vi "SetStringValue.vi"(8 "error in (no error)":errorcluster caption="错误输入（无错误）", 9 "strValue":string, 10 "strKey":string, 11 "handle":u64) -> (0 "error out":errorcluster caption="错误输出", 1 "strValue":string, 2 "function return":i32, 3 "handle out":u64)   [LabVIEW 2015, in "MvCameraControl.lvlib"]
doc: "MV_LV_API int __stdcall GetStringValue( void* handle, const char* strKey, MVCC_STRINGVALUE *pStringValue);"
uses:
  MvCameraControl.lvlib
  MvCameraControl.dll
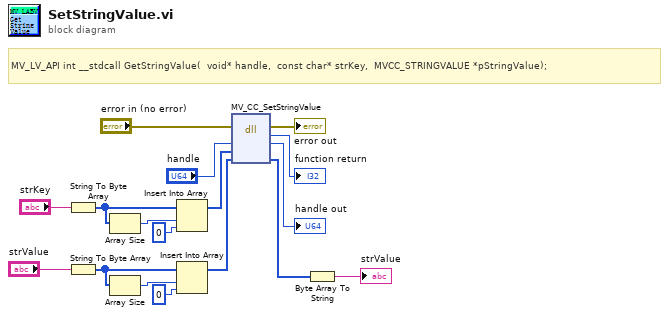
[diagram p0: block diagram]
diagram:
  # "MV_LV_API int __stdcall GetStringValue(  void* handle,  const char* strKey,  MVCC_STRINGVALUE *pStringValue);"
  n1 = String To Byte Array(string="strKey") -> (unsigned byte array=w13:u8[])
  n2 = String To Byte Array(string="strValue") -> (unsigned byte array=w8:u8[])
  n3 = Array Size(array=w13) -> (size(s)=w12:i32)
  n4 = Array Size(array=w8) -> (size(s)=w7:i32)
  n5 = Insert Into Array(array=w13, index=w12, new element=u8 0 ("新元素/子数组")) -> (w9:u8[])
  n6 = Insert Into Array(array=w8, index=w7, new element=u8 0 ("新元素/子数组")) -> (w4:u8[])
  n7 = dll-call lib="MvCameraControl.dll" fn="MV_CC_SetStringValue"(error in="error in (no error)", "handle"="handle", "strKey"=w9, "pStringValue"=w4) -> (error out=→"error out":errorcluster, "返回类型"=→"function return":i32, "handle"=→"handle out":u64, "pStringValue"=w3:u8[])  [unwired: 3 in, 1 out]
  n8 = Byte Array To String(unsigned byte array=w3) -> (string=→"strValue":string)
